vi "DOCK_listbox_set_values_and_recolor.vi"(7 "column_names":string[](array[string]), 8 "error_in":errorcluster, 10 "REPORT_GEAR_station":T1=12 caption="Station:" items=["ALL"=0, "Station 10"=10, "Station 20"=20, "Station 30"=30, "Station 40"=40, "Station 50"=50, "Station 60"=60, "Station 70"=70, "Station 80"=80, "Station 90"=90, "Station 100"=100, "Station 110"=110, "Station 120"=120, "Station 160"=165], 11 "REPORT_all_info":T2) -> (0 "error_out":errorcluster)   [LabVIEW 2019]
uses:
  DOCK_all_info.ctl
  DOCK_reference_data.ctl
  MAIN/DOCK_header_data_display.ctl
  DOCK_gear_statuses.ctl
  DOCK_references.ctl
  DOCK_gear_station.ctl
  <vilib>/Utility/miscctls.llb/LVRowAndColumnTypeDef.ctl
  <vilib>/Utility/miscctls.llb/LVRowAndColumnUnsignedTypeDef.ctl
  <userlib>/_OpenG.lib/array/array.llb/Filter 1D Array with Scalar (String)__ogtk.vi
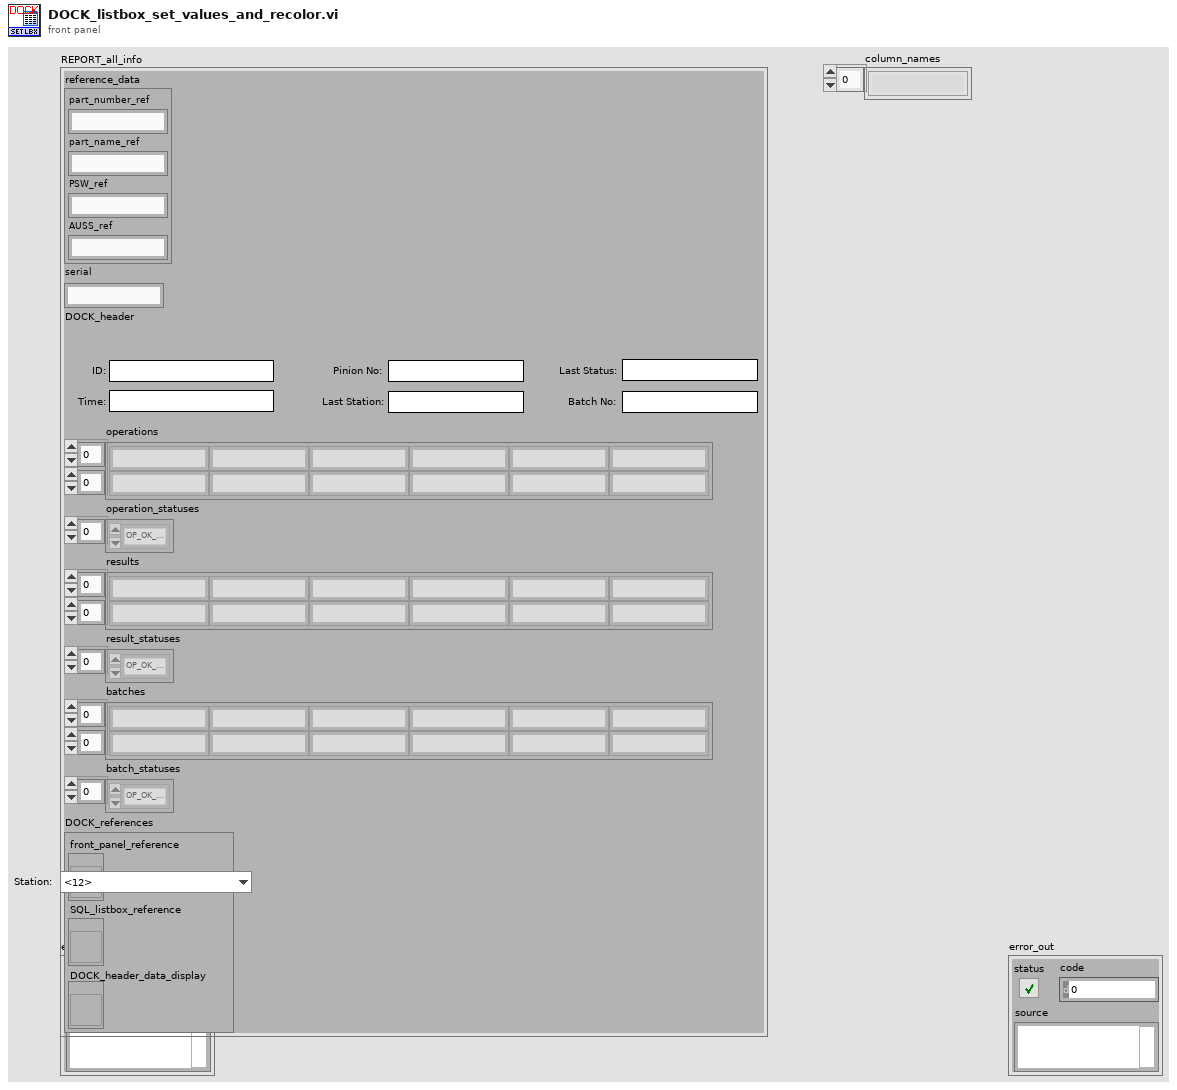
[diagram p1: front panel]
types:
  T1 = typedef "DOCK_gear_station.ctl" = u16
  T2 = typedef "DOCK_all_info.ctl" = cluster{"reference_data":T3, "serial":string, "DOCK_header":T4, "operations":string[][], "operation_statuses":T5[], "results":string[][], "result_statuses":T5[], "batches":string[][], "batch_statuses":T5[], "DOCK_references":T6}
  T3 = typedef "DOCK_reference_data.ctl" = cluster{"part_number_ref":string, "part_name_ref":string, "PSW_ref":string, "AUSS_ref":string}
  T4 = typedef "DOCK_header_data_display.ctl" = cluster{"ID":string, "creation_time":string, "last_station":string, "last_status":string, "pinion_serial":string, "batch_code":string}
  T5 = typedef "DOCK_GEAR_statuses.ctl" = enum16{"OP_OK_hide", "OP_OK_show", "OP_NOK_hide", "OP_NOK_show", "OP_interrupted_hide", "OP_interrupted_show", "OP_in_operation_hide", "OP_in_operation_show", "OP_unexpected_hide", "OP_unexpected_show", "RE_REAL_OK", "RE_REAL_NOK", "RE_STRING", "RE_sub_header", "RE_no_data", "RE_unexpected", "BA_sub_header", "BA_data", "BA_no_data"}
  T6 = typedef "DOCK_references.ctl" = cluster{"front_panel_reference":refnum<vi>, "SQL_listbox_reference":refnum<vi>, "DOCK_header_data_display":refnum<vi>}
  T7 = typedef "LVRowAndColumnUnsignedTypeDef.ctl" = cluster{"Row":u32, "Column":u32}
  T8 = typedef "LVRowAndColumnTypeDef.ctl" = cluster{"Row":i32, "Column":i32}
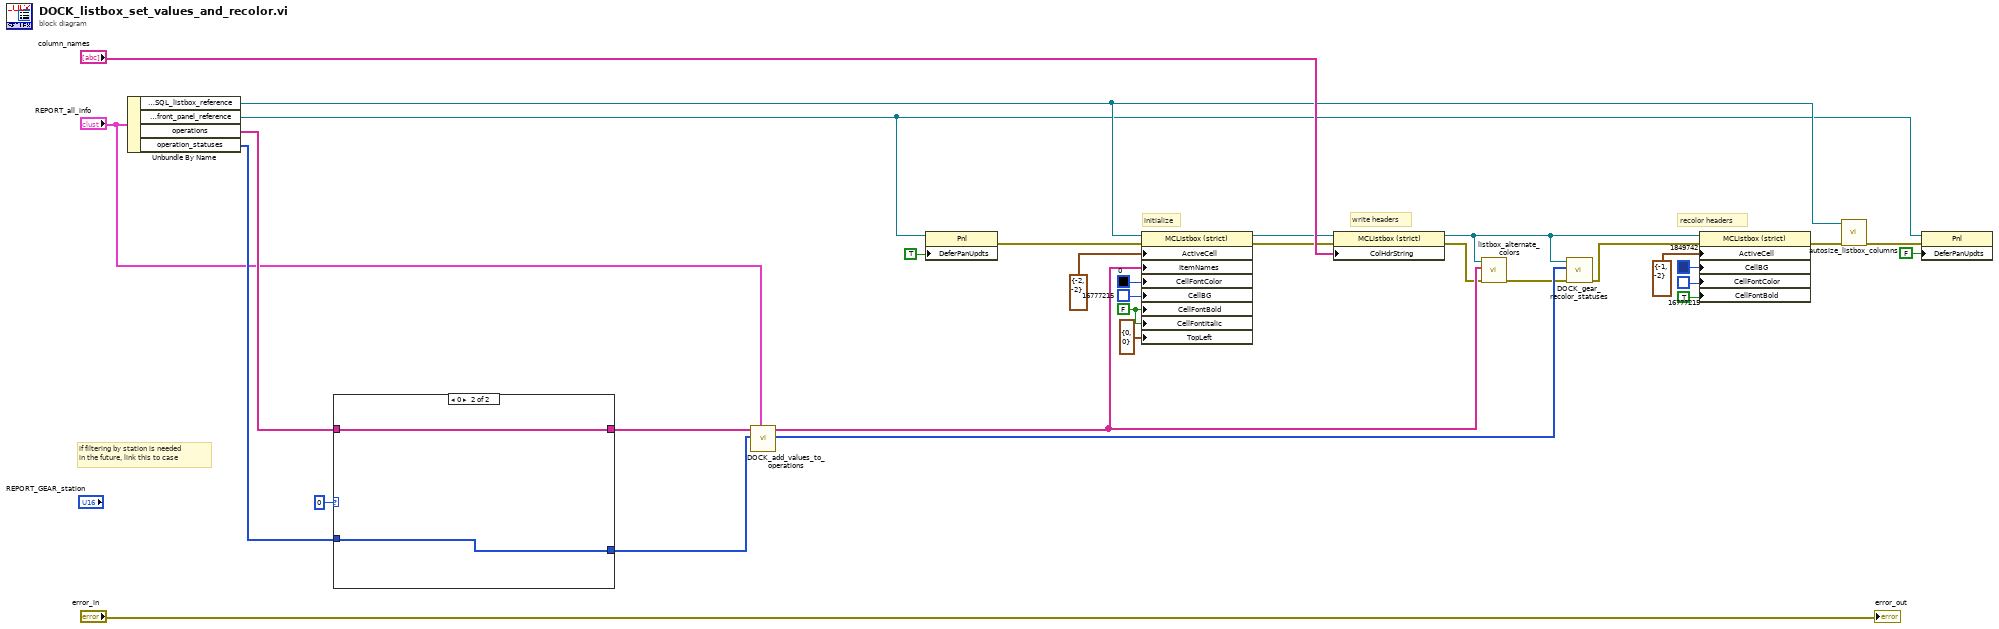
[diagram p0: block diagram]
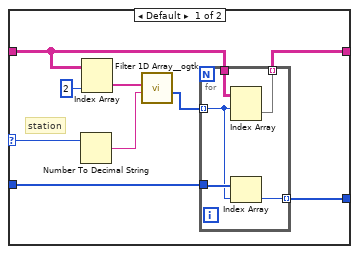
[diagram p2: hidden frame]
diagram:
  w16 = FALSE ("Active Cell:Cell Font:Bold")
  # "if filtering by station is needed\nin the future, link this to case"
  # "recolor headers"
  # "initialize"
  # "write headers"
  n1 = Unbundle By Name("REPORT_all_info") -> ("DOCK_references.SQL_listbox_reference"=w23:refnum<vi>, "DOCK_references.front_panel_reference"=w22:refnum<vi>, "operations"=w21:string[][], "operation_statuses"=w20:T5[])
  n2 = case shown="0" 0 {
    selector: 0 -> [w36 _]
    tunnel: w21 -> [w39 w48]
    tunnel: [w37 w48] -> w19
    tunnel: w20 -> [w34 w47]
    tunnel: [w33 w47] -> w18
    frame Default {
      # "station"
      n3 = Number To Decimal String(number=w36) -> (decimal integer string=w35:string)  [unwired: 1 in]
      n4 = Index Array(array=w39, index (col)=2 ("disabled index (col)")) -> (element=w40:string[])  [unwired: 1 in]
      n5 = call-poly <userlib>:"Filter 1D Array__ogtk.vi"("items to filter"=w35, "array"=w40) -> ("filtered item indices"=w38:i32[])  [unwired: 4 in, 1 out]
      n6 = for {
        tunnel: w39 -> [w46]
        tunnel: w38 -> [w43] mode=indexing
        tunnel: [w45] -> w37 mode=indexing
        tunnel: w34 -> [w44]
        tunnel: [w42] -> w33 mode=indexing
        n7 = Index Array(array=w46, index (row)=w43) -> (element=w45:string[])  [unwired: 1 in]
        n8 = Index Array(array=w44, index=w43) -> (element=w42:T5)
      }
    }
    frame 0 {
    }
  }
  n9 = call "DOCK_add_values_to_operations.vi"("REPORT_all_info"="REPORT_all_info", "operation_statuses"=w18, "operations"=w19) -> ("record_statuses"=w7:T5[], "ItemNames"=w13:string[][])  [unwired: 7 in]
  n10 = property on="Property Node" class="Pnl"(reference=w22, "DeferPanUpdts"=TRUE ("Defer Panel Updates")) -> (error out=w30:errorcluster)  [unwired: 1 in, 1 out]
  n11 = property on="Property Node" class="MCListbox (strict)"(reference=w23, error in=w30, "ActiveCell"=T8 {"Row"=-2, "Column"=-2} ("Active Cell:Active Cell"), "ItemNames"=w13, "CellFontColor"=u32 0, "CellBG"=u32 16777215, "CellFontBold"=w16, "CellFontItalic"=w16, "TopLeft"=T7 {"Row"=0, "Column"=0} ("Top Left Visible Cell")) -> (reference out=w26:refnum<vi>, error out=w24:errorcluster)
  n12 = property on="Property Node" class="MCListbox (strict)"(reference=w26, error in=w24, "ColHdrString"="column_names") -> (reference out=w8:refnum<vi>, error out=w5:errorcluster)
  n13 = call "listbox_alternate_colors.vi"("error_in"=w5, "item_names"=w13, "listbox_ref"=w8) -> ("error_out"=w6:errorcluster)  [unwired: 8 in]
  n14 = call "DOCK_gear_recolor_statuses.vi"("error_in"=w6, "record_statuses"=w7, "listbox_ref"=w8) -> ("error_out"=w4:errorcluster)  [unwired: 8 in]
  n15 = property on="Property Node" class="MCListbox (strict)"(reference=w8, error in=w4, "ActiveCell"=T8 {"Row"=-1, "Column"=-2} ("Active Cell:Active Cell"), "CellBG"=u32 1849742, "CellFontColor"=u32 16777215, "CellFontBold"=TRUE ("Active Cell:Cell Font:Bold")) -> (error out=w29:errorcluster)  [unwired: 1 out]
  n16 = call "autosize_listbox_columns.vi"("error in (no error)"=w29, "Table Ref"=w23) -> ("error out"=w28:errorcluster)  [unwired: 4 in, 1 out]
  n17 = property on="Property Node" class="Pnl"(reference=w22, error in=w28, "DeferPanUpdts"=FALSE ("Defer Panel Updates")) -> ()  [unwired: 2 out]
  "error_out" <- "error_in"
